vi "P612_Init.vi"() -> (1 "Status":bool, 2 "Position":dbl[](array[numeric]), 3 "VISA Refnum out":refnum<visa-resource-name>)   [LabVIEW 2014]
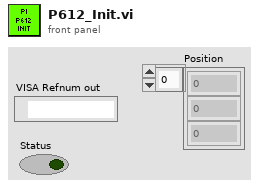
[diagram p1: front panel]
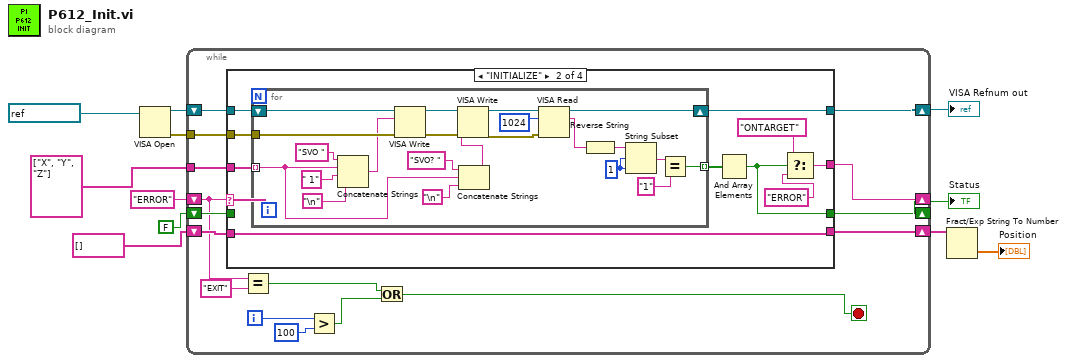
[diagram p0: block diagram]
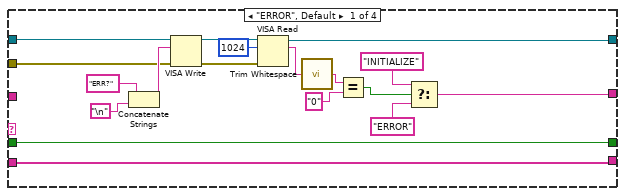
[diagram p2: hidden frame]
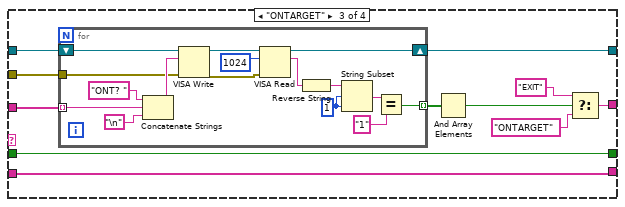
[diagram p3: hidden frame]
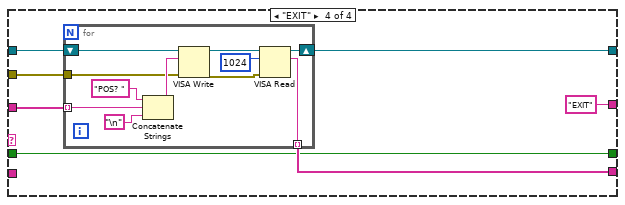
[diagram p4: hidden frame]
diagram:
  n1 = VISA Open(VISA resource name=refnum<visa-resource-name> "PI_E-816") -> (VISA resource name=w10:refnum<visa-resource-name>, error out=w9:errorcluster)  [unwired: 4 in]
  n2 = while {
    tunnel: w9 -> [w25]
    shift-right: [w24] -> _
    shift-left: "ERROR" ("string") -> [w16]
    shift-right: [w27] -> w11
    shift-left: FALSE -> [w21]
    shift-right: [w22] -> w2
    shift-left: string[] [] ("read buffer") -> [w20]
    shift-right: [w23] -> w6
    shift-left: w10 -> [w26]
    tunnel: string[] ["X", "Y", "Z"] -> [w12]
    i -> [w19]
    stop <- w14 stop-if-true
    n3 = case shown="\"INITIALIZE\"" w16 {
      tunnel: [w28 w46 w81 w106] -> w27
      tunnel: w26 -> [w41 w55 w84 w111]
      tunnel: w25 -> [w39 w54 w83 w110]
      tunnel: [w31 w53 w88 "EXIT" ("string")] -> w24
      tunnel: [w30 w48 w82 w107] -> w23
      tunnel: [w29 w49 w80 w108] -> w22
      tunnel: w21 -> [w28 _ w81 w106]
      tunnel: w20 -> [w29 w49 w80 _]
      tunnel: w12 -> [_ w47 w78 w105]
      frame "ERROR", Default {
        n4 = Concatenate Strings("ERR?" ("string"), "\n") -> (w44:string)
        n5 = VISA Write(VISA resource name=w41, write buffer=w44, error in (no error)=w39) -> (VISA resource name out=w45:refnum<visa-resource-name>, error out=w38:errorcluster)  [unwired: 1 out]
        n6 = VISA Read(VISA resource name=w45, byte count=u32 1024, error in (no error)=w38) -> (VISA resource name out=w30:refnum<visa-resource-name>, read buffer=w37:string)  [unwired: 2 out]
        n7 = call <vilib>:"Trim Whitespace.vi"("string"=w37) -> ("trimmed string"=w35:string)  [unwired: 1 in]
        n8 = Equal?(x=w35, y="0") -> (x = y?=w34:bool)
        n9 = Select(t="INITIALIZE", s=w34, f="ERROR" ("string")) -> (s? t:f=w31:string)
      }
      frame "INITIALIZE" {
        n10 = for {
          tunnel: w54 -> [w76]
          tunnel: [w72] -> w50 mode=indexing
          tunnel: w47 -> [w56] mode=indexing
          shift-right: [w71] -> w48
          shift-left: w55 -> [w77]
          w60 = 1 ("length (rest)")
          n11 = Concatenate Strings("SVO " ("string"), w56, " 1" ("string"), "\n") -> (w64:string)
          n12 = VISA Write(VISA resource name=w77, write buffer=w64, error in (no error)=w76) -> (VISA resource name out=w74:refnum<visa-resource-name>, error out=w73:errorcluster)  [unwired: 1 out]
          n13 = Concatenate Strings("SVO? " ("string"), w56, "\n") -> (w69:string)
          n14 = VISA Write(VISA resource name=w74, write buffer=w69, error in (no error)=w73) -> (VISA resource name out=w67:refnum<visa-resource-name>, error out=w66:errorcluster)  [unwired: 1 out]
          n15 = VISA Read(VISA resource name=w67, byte count=u32 1024, error in (no error)=w66) -> (VISA resource name out=w71:refnum<visa-resource-name>, read buffer=w75:string)  [unwired: 2 out]
          n16 = Reverse String(1:w75) -> (0:w61:string)
          n17 = String Subset(string=w61, offset (0)=w60, length (rest)=w60) -> (substring=w59:string)
          n18 = Equal?(x=w59, y="1") -> (x = y?=w72:bool)
        }
        n19 = And Array Elements(Boolean array=w50) -> (logical AND=w46:bool)
        n20 = Select(t="ONTARGET" ("string"), s=w46, f="ERROR" ("string")) -> (s? t:f=w53:string)
      }
      frame "ONTARGET" {
        n21 = for {
          tunnel: [w94] -> w85 mode=indexing
          tunnel: w83 -> [w92]
          shift-right: [w91] -> w82
          shift-left: w84 -> [w93]
          tunnel: w78 -> [w89] mode=indexing
          w100 = 1 ("length (rest)")
          n22 = Concatenate Strings("ONT? " ("string"), w89, "\n") -> (w103:string)
          n23 = VISA Write(VISA resource name=w93, write buffer=w103, error in (no error)=w92) -> (VISA resource name out=w96:refnum<visa-resource-name>, error out=w95:errorcluster)  [unwired: 1 out]
          n24 = VISA Read(VISA resource name=w96, byte count=u32 1024, error in (no error)=w95) -> (VISA resource name out=w91:refnum<visa-resource-name>, read buffer=w99:string)  [unwired: 2 out]
          n25 = Reverse String(1:w99) -> (0:w101:string)
          n26 = String Subset(string=w101, offset (0)=w100, length (rest)=w100) -> (substring=w98:string)
          n27 = Equal?(x=w98, y="1") -> (x = y?=w94:bool)
        }
        n28 = And Array Elements(Boolean array=w85) -> (logical AND=w79:bool)
        n29 = Select(t="EXIT" ("string"), s=w79, f="ONTARGET" ("string")) -> (s? t:f=w88:string)
      }
      frame "EXIT" {
        n30 = for {
          tunnel: w110 -> [w116]
          tunnel: [w115] -> w108 mode=indexing
          shift-right: [w114] -> w107
          shift-left: w111 -> [w117]
          tunnel: w105 -> [w112] mode=indexing
          n31 = Concatenate Strings("POS? " ("string"), w112, "\n") -> (w121:string)
          n32 = VISA Write(VISA resource name=w117, write buffer=w121, error in (no error)=w116) -> (VISA resource name out=w119:refnum<visa-resource-name>, error out=w118:errorcluster)  [unwired: 1 out]
          n33 = VISA Read(VISA resource name=w119, byte count=u32 1024, error in (no error)=w118) -> (VISA resource name out=w114:refnum<visa-resource-name>, read buffer=w115:string)  [unwired: 2 out]
        }
      }
    }
    n34 = Equal?(x=w16, y="EXIT") -> (x = y?=w15:bool)
    n35 = Greater?(x=w19, y=100 ("x")) -> (0:w17:bool)
    n36 = Or(x=w15, y=w17) -> (x .or. y?=w14:bool)
  }
  "Status" <- w11
  "VISA Refnum out" <- w6
  n37 = Fract/Exp String To Number(string=w2) -> (number=→"Position":dbl[])  [unwired: 3 in, 1 out]
